vi "New Component Loader Error.vi"(7 "error source vi name":string, 11 "error":T1) -> (1 "new offset":i32, 3 "error out":errorcluster)   [LabVIEW 2017, in "DSF Core.lvlib" / "Component Loader.lvclass"]
uses:
  Component Loader.lvclass
  Errors.ctl
  <vilib>/NI/Memory Manager/VIs/New Error Cluster (512B).vi
  VIs/Constants/Engine Library Name.vi
  <vilib>/NI/Memory Manager/Static Errors.lvlib
  Framework/Framework.lvclass
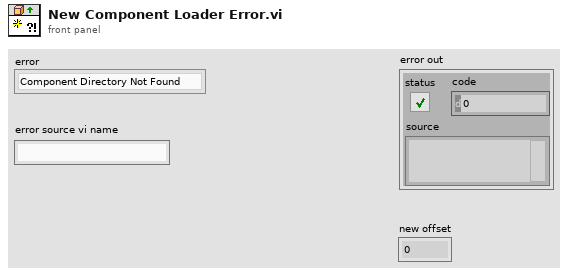
[diagram p1: front panel]
types:
  T1 = typedef "DSF Core.lvlib/Component Loader.lvclass/Errors.ctl" = enum16{"Component Directory Not Found", "Component Not Found", "Class Not Found"}
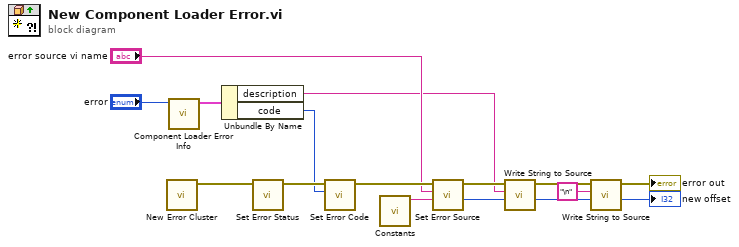
[diagram p0: block diagram]
diagram:
  n1 = call-poly <vilib>:"New Error Cluster.vi"() -> ("error out"=w15:errorcluster)  [unwired: 10 in, 1 out]
  n2 = call "Component Loader Error Info.vi"("error"="error") -> ("error info"=w13:cluster{"code":i32, "description":string})  [unwired: 10 in]
  n3 = Unbundle By Name(w13) -> ("description"=w6:string, "code"=w12:i32)
  n4 = call <vilib>:"Set Error Status.vi"("error in"=w15) -> ("error out"=w14:errorcluster)  [unwired: 9 in, 1 out]
  n5 = call <vilib>:"Set Error Code.vi"("code"=w12, "error in"=w14) -> ("error out"=w11:errorcluster)  [unwired: 8 in, 1 out]
  n6 = call-poly "Constants.vi"() -> ("Engine Library Name"=w9:string)  [unwired: 11 in]
  n7 = call <vilib>:"Set Error Source.vi"("library name (\"\")"=w9, "vi name"="error source vi name", "error in"=w11) -> ("initial offset"=w7:i32, "error out"=w8:errorcluster)  [unwired: 7 in]
  n8 = call <vilib>:"Write String to Source.vi"("offset"=w7, "string"=w6, "error in"=w8) -> ("new offset"=w3:i32, "error out"=w5:errorcluster)  [unwired: 7 in]
  n9 = call <vilib>:"Write String to Source.vi"("offset"=w3, "string"="\n", "error in"=w5) -> ("new offset"=→"new offset":i32, "error out"=→"error out":errorcluster)  [unwired: 7 in]
